vi "Create from SSH.vi"(8 "Error In":errorcluster, 11 "SSH":refnum<class "SSH.lvclass">) -> (0 "Error Out":errorcluster, 3 "File Info":refnum<class "File Info.lvclass">)   [LabVIEW 2021, in "Field_RnD_Services_LIBSSH2_Toolkit.lvlib" / "File Info.lvclass"]
doc: "Creates a new File Info object from a SSH context."
uses:
  File Info.lvclass
  SSH/SSH.lvclass
  File Info.lvclass/File Info.ctl
  Field_RnD_Services_LIBSSH2_Toolkit.lvlib
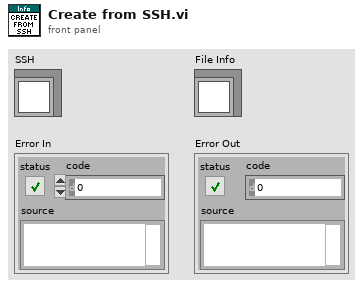
[diagram p1: front panel]
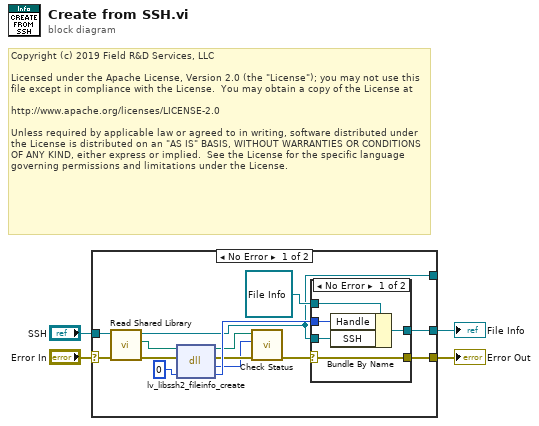
[diagram p0: block diagram]
diagram:
  # "Copyright (c) 2019 Field R&D Services, LLC\n\nLicensed under the Apache License, Version 2.0 (the \"License\"); you may not use this file except in compliance with the License.  You may obtain a copy of the License at\n\nhttp://www.apache.org/licenses/LICENSE-2.0\n\nUnless required by applicable law or agreed to in writing, software distributed under the License is distributed on an \"AS IS\" BASIS, WITHOUT WARRANTIES OR CONDITIONS OF ANY KIND, either express or implied.  See the License for the specific language governing permissions and limitations under the License."
  n1 = case shown="No Error" "Error In" {
    selector: "Error In" -> [w9 w27]
    tunnel: [w11 w27] -> w3
    tunnel: [w18 _] -> w2
    tunnel: "SSH" -> [w10 w26]
    tunnel: [w5 w26] -> _
    frame No Error {
      n2 = call "Read Shared Library.vi"("Error In"=w9, "SSH In"=w10) -> ("Error Out"=w8:errorcluster, "libssh2lv Shared Library"=w7:path, "SSH Out"=w5:refnum<class "SSH.lvclass">)  [unwired: 7 in]
      n3 = dll-call lib="lv-libssh2.*" fn="lv_libssh2_fileinfo_create"(path in=w7, error in=w8, "handle"=u64 0) -> (path out=w14:path, error out=w15:errorcluster, "status"=w13:i32, "handle"=w16:u64)  [unwired: 1 in]
      n4 = call "Check Status.vi"("Error In"=w15, "Status"=w13, "libssh2lv Shared Library In"=w14) -> ("Error Out"=w12:errorcluster)  [unwired: 7 in, 1 out]
      n5 = case shown="No Error" w12 {
        selector: w12 -> [w21 w25]
        tunnel: [w23 w24] -> w18
        tunnel: w16 -> [w22 _]
        tunnel: [w21 w25] -> w11
        tunnel: w5 -> [w20 _]
        tunnel: refnum<class "File Info.lvclass"> refnum ("Toolkit.lvlib:SFTP Attributes.lvclass") -> [w19 w24]
        frame No Error {
          n6 = Bundle By Name(cluster=w19, "Handle"=w22, "SSH"=w20) -> (w23:refnum<class "File Info.lvclass">)
        }
        frame Error {
        }
      }
    }
    frame Error {
    }
  }
  "Error Out" <- w3
  "File Info" <- w2
